vi "sensor-SubVI.vi"(2 "stop 2":bool, 3 "Number of Samples to Read":i32=100, 5 "Sample Rate":dbl=1000.0) -> (0 "Distance":dbl(knob) scale=10.0..20.0, 1 "Filter":dynamicdata(graph), 4 "Distance \n 2":dbl, 6 "Mean":dbl(graph), 7 "Voltage":dbl, 8 "Result":dbl, 9 "Signal":dynamicdata(graph))   [LabVIEW 2010]
uses:
  <vilib>/express/express arith-compare/Formula/XNode/ExpressFormulaBlockNode.xnode
  <vilib>/Analysis/NI_AALBase.lvlib
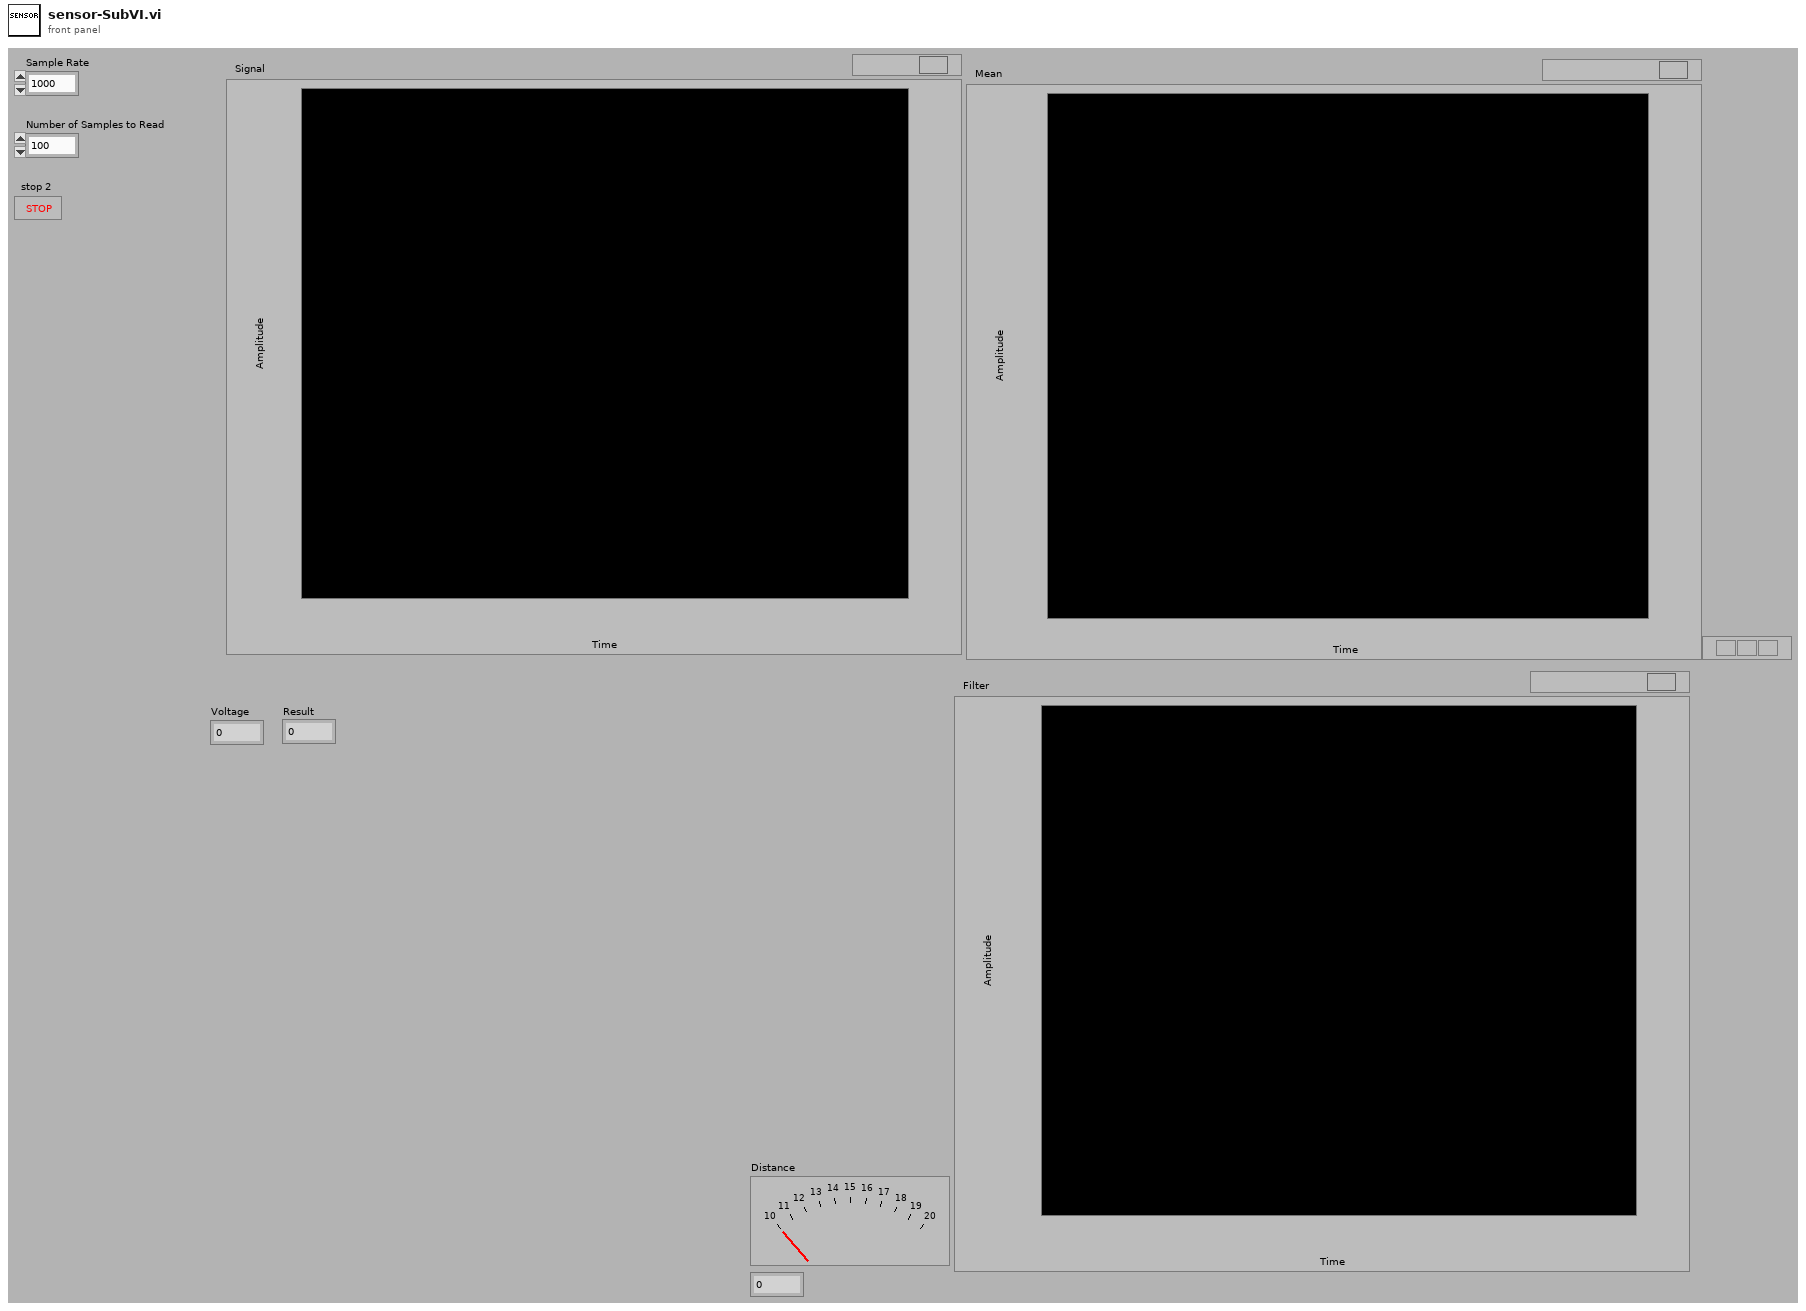
[diagram p1: front panel]
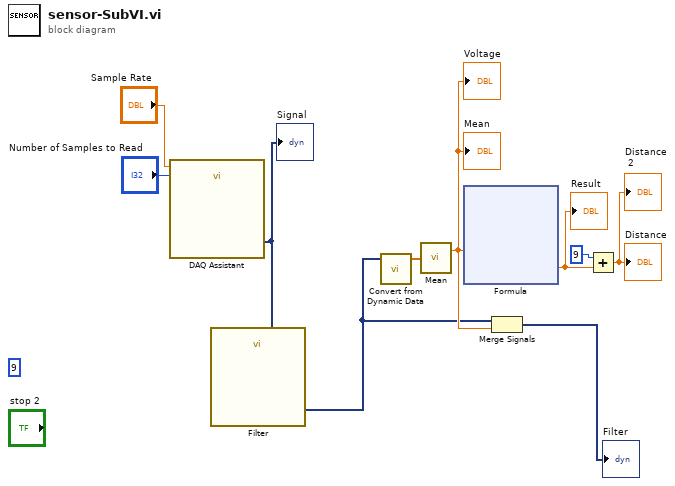
[diagram p0: block diagram]
diagram:
  (unwired) 9
  n1 = call "DAQ Assistant"("rate"="Sample Rate", "number of samples"="Number of Samples to Read") -> ("data"=w4:dynamicdata)  [unwired: 14 in, 3 out]
  "Signal" <- w4
  n2 = call "Filter"("Signal"=w4) -> ("Filtered Signal"=w2:dynamicdata)  [unwired: 9 in, 1 out]
  n3 = call "Convert from Dynamic Data"("Dynamic Data Type"=w2) -> ("Array"=w7:dbl[])  [unwired: 3 in]
  n4 = call <vilib>:"Mean.vi"("X"=w7) -> ("mean"=w3:dbl)  [unwired: 1 out]
  "Mean" <- w3
  "Voltage" <- w3
  n5 = xnode "Formula"("X1"=w3) -> ("Result"=w9:dbl)  [unwired: 1 in, 1 out]
  "Result" <- w9
  n6 = Merge Signals(w2, w3) -> (→"Filter":dynamicdata)
  n7 = Add(x=9, y=w9) -> (x+y=→"Distance" →"Distance \n 2":dbl)
